vi "MagazineStateController.vi"(1 "Selected State (In)":string) -> (0 "Selected State (Out)":string)   [LabVIEW 2019]
uses:
  dsinstructions.vi
  outputs.vi
panel:
  in  "Magazine_Reverse_Power":dbl=-0.7 format="%#_13g"
  in  "Flapper_Period_Down (ms)":u32=200
  in  "Flapper_Period_Total (ms)":u32=1000
  in  "Magazine_Power":dbl=0.7 format="%#_13g"
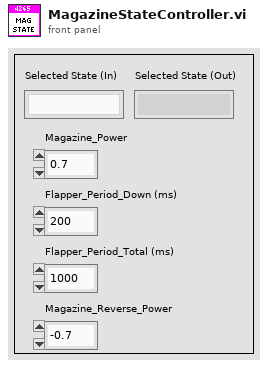
[diagram p1: front panel]
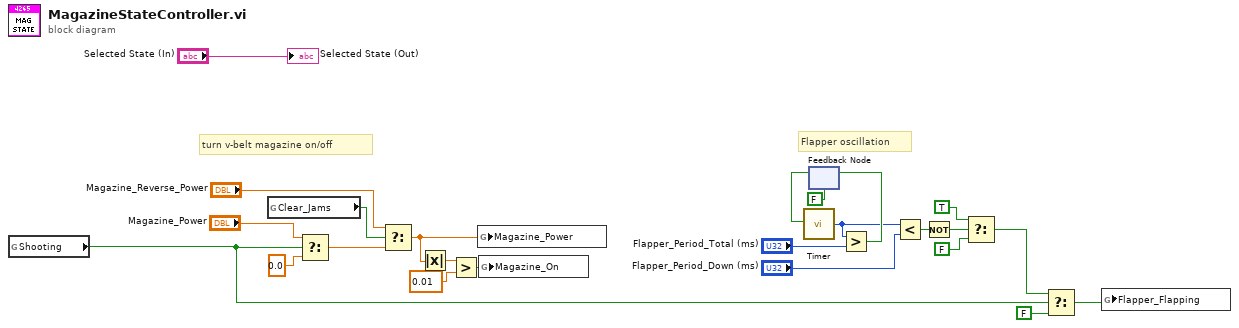
[diagram p0: block diagram]
diagram:
  # "Flapper oscillation"
  # "turn v-belt magazine on/off"
  n1 = global read "outputs.vi" "Shooting"() -> (w8:bool)
  n2 = global read "dsinstructions.vi" "Clear_Jams"() -> (w24:bool)
  n3 = Select(t="Magazine_Power", s=w8, f=0.0) -> (s? t:f=w22:dbl)
  n4 = Select(t="Magazine_Reverse_Power", s=w24, f=w22) -> (s? t:f=w6:dbl)
  n5 = Absolute Value(x=w6) -> (abs(x)=w5:dbl)
  n6 = Greater?(x=w5, y=0.01) -> (0:w3:bool)
  n7 = global write "outputs.vi" "Magazine_Power"(w6) -> ()
  n8 = global write "outputs.vi" "Magazine_On"(w3) -> ()
  n9 = feedback #1(FALSE) -> (w2:bool)
  n10 = call "Timer.vi"("Reset Timer"=w2) -> ("Time (ms)"=w1:u32)
  n11 = Greater?(x=w1, y="Flapper_Period_Total (ms)") -> (0:w16:bool)
  n12 = feedback-in #1(w16) -> ()
  n13 = Less?(x=w1, y="Flapper_Period_Down (ms)") -> (x < y?=w19:bool)
  n14 = Not(x=w19) -> (.not. x?=w20:bool)
  n15 = Select(t=TRUE, s=w20, f=FALSE) -> (s? t:f=w21:bool)
  n16 = Select(t=w21, s=w8, f=FALSE) -> (s? t:f=w12:bool)
  n17 = global write "outputs.vi" "Flapper_Flapping"(w12) -> ()
  "Selected State (Out)" <- "Selected State (In)"
